vi "Message Log.vi"(8 "error in":errorcluster, 10 "close?":bool, 11 "Message":string) -> (0 "error out":errorcluster)   [LabVIEW 2012]
uses:
  Reusable/File IO/File Utilities.lvlib
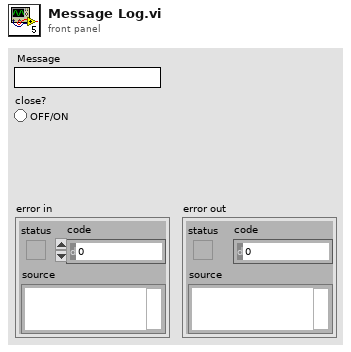
[diagram p1: front panel]
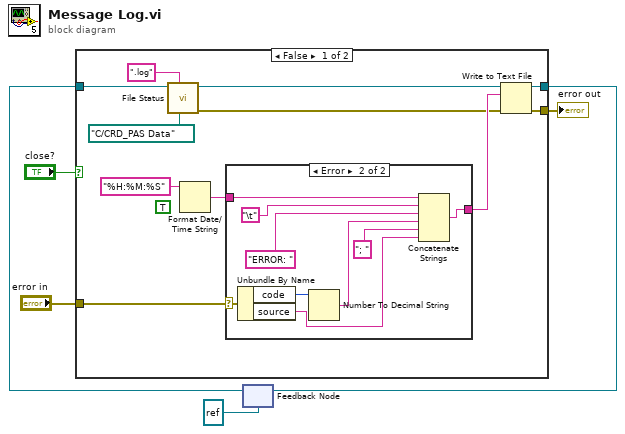
[diagram p0: block diagram]
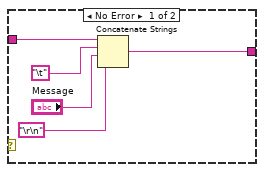
[diagram p2: hidden frame]
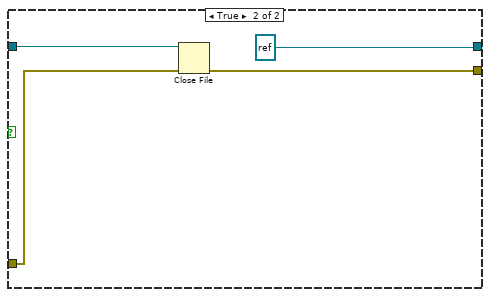
[diagram p3: hidden frame]
diagram:
  n1 = feedback #1(refnum<file> refnum ("fileRefOut")) -> (w3:refnum<file>)
  n2 = case shown="False" "close?" {
    tunnel: "error in" -> [w13 w33]
    tunnel: [w12 w32] -> w5
    tunnel: w3 -> [w8 w34]
    tunnel: [w7 refnum<file> refnum ("refnum out")] -> w2
    frame False {
      (unwired) TRUE ("UTC format")
      n3 = call "File Status.vi"("Data Path"=path "C:/CRD_PAS Data", "ext"=".log", "fileRefIn"=w8) -> ("error out"=w11:errorcluster, "fileRefOut"=w14:refnum<file>)  [unwired: 7 in]
      n4 = Format Date/Time String(time format string (%c)="%H:%M:%S") -> (date/time string=w9:string)  [unwired: 2 in]
      n5 = case shown="Error" w13 {
        selector: w13 -> [_ w28]
        tunnel: [w19 w23] -> w15
        tunnel: w9 -> [w18 w31]
        frame No Error {
          n6 = Concatenate Strings(w18, "\t", "Message", "\r\n") -> (w19:string)
        }
        frame Error {
          n7 = Unbundle By Name(w28) -> ("code"=w27:i32, "source"=w24:string)
          n8 = Number To Decimal String(number=w27) -> (decimal integer string=w26:string)  [unwired: 1 in]
          n9 = Concatenate Strings(w31, "\t", "ERROR: " ("string"), w26, "; " ("string"), w24) -> (w23:string)
        }
      }
      n10 = Write to Text File(file (use dialog)=w14, text=w15, error in=w11) -> (refnum out=w7:refnum<file>, error out=w12:errorcluster)  [unwired: 1 in, 1 out]
    }
    frame True {
      n11 = Close File(refnum=w34, error in=w33) -> (error out=w32:errorcluster)  [unwired: 1 out]
    }
  }
  "error out" <- w5
  n12 = feedback-in #1(w2) -> ()
